vi "From Variant.vi"(0 "Derived in":refnum<class "KDemoBase.lvclass">, 7 "Variant":variant, 9 "Prefix":string="Derived", 11 "error in (no error)":errorcluster) -> (4 "Derived out":refnum<class "KDemoBase.lvclass">, 15 "error out":errorcluster)   [LabVIEW 2015, in "KDemoBase.lvclass"]
uses:
  KDemoBase.lvclass
  KDemoBase.lvclass/KDemoBase.ctl
  KObject Class/KObject.lvclass
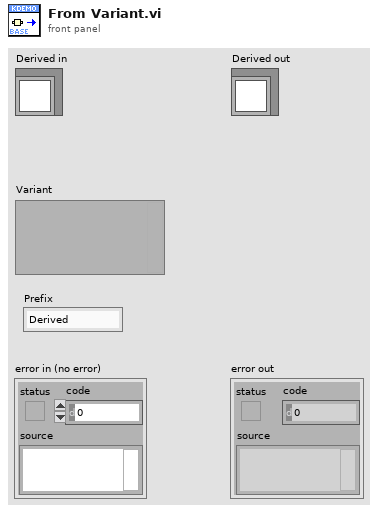
[diagram p1: front panel]
types:
  T1 = typedef "KDemoBase.lvclass/Serialized.ctl" = cluster{"Boolean":bool, "Value":dbl}
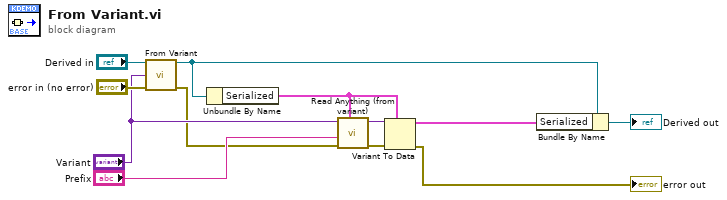
[diagram p0: block diagram]
diagram:
  n1 = call-parent "From Variant.vi"("KObject in"="Derived in", "Variant"="Variant", "error in (no error)"="error in (no error)") -> ("KObject out"=w9:refnum<class "KDemoBase.lvclass">, "error out"=w4:errorcluster)  [unwired: 11 in]
  n2 = Unbundle By Name(w9) -> ("Serialized"=w8:T1)
  n3 = call "Read Anything (from variant).vi"("Type of Anything"=w8, "Error In"=w4, "Prefix"="Prefix", "Variant Database"="Variant") -> ("Error Out"=w7:errorcluster, "Anything"=w6:variant)  [unwired: 5 in, 1 out]
  n4 = Variant To Data(error in=w7, type=w8, Variant=w6) -> (data=w1:T1, error out=→"error out":errorcluster)
  n5 = Bundle By Name(cluster=w9, "Serialized"=w1) -> (→"Derived out":refnum<class "KDemoBase.lvclass">)
